vi "Identify Control Index.vi"(11 "control ref":refnum<vi>) -> (3 "index":i32)   [LabVIEW 2023]
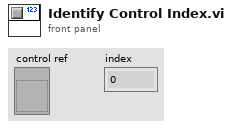
[diagram p1: front panel]
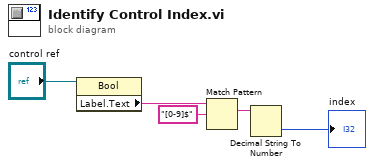
[diagram p0: block diagram]
diagram:
  n1 = property class="Bool"(reference="control ref") -> ("Label.Text"=w2:string)  [unwired: 1 in, 2 out]
  n2 = Match Pattern(string=w2, regular expression="[0-9]$") -> (match substring=w4:string)  [unwired: 1 in, 3 out]
  n3 = Decimal String To Number(string=w4) -> (number=→"index":i32)  [unwired: 2 in, 1 out]
